vi "Check FETs (Debug).vi"() -> ()   [LabVIEW 2009]
panel:
  out "Debug":string
  out "Emergency Stop":bool=TRUE
  out "Input E":bool=TRUE
  out "Motors on?":bool=TRUE
  out "MC Init Complete":bool=TRUE
  in  "MC VISA resource in":refnum<visa-resource-name>="ASRL1::INSTR"
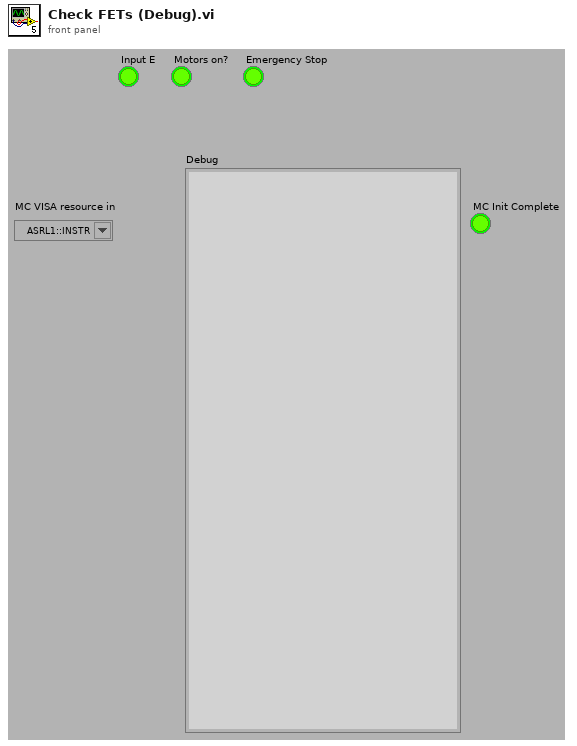
[diagram p1: front panel]
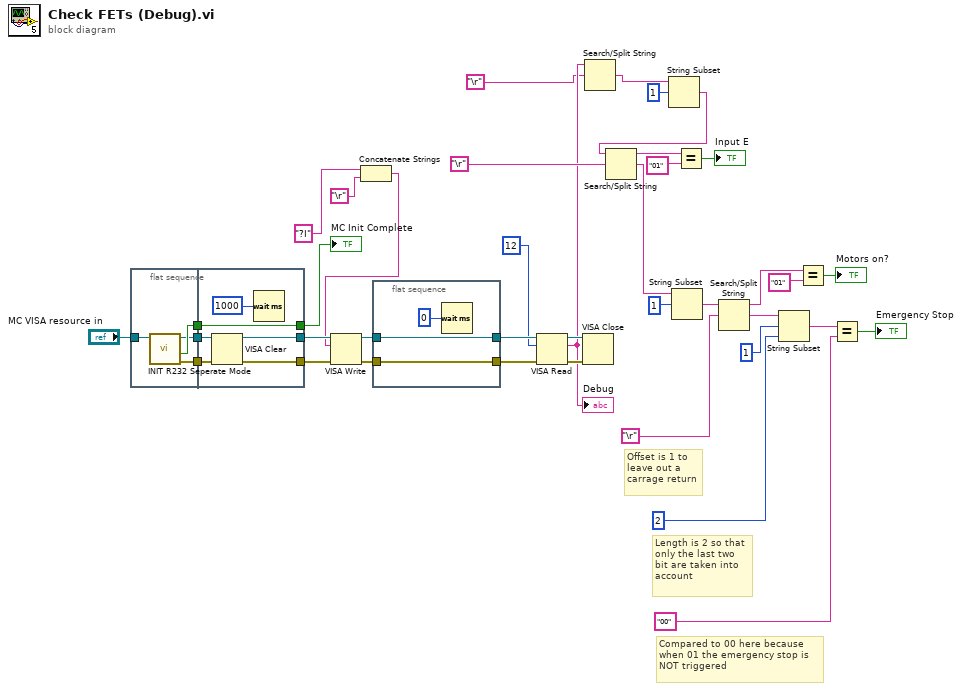
[diagram p0: block diagram]
diagram:
  # "Compared to 00 here because\nwhen 01 the emergency stop is\nNOT triggered"
  # "Length is 2 so that\nonly the last two\nbit are taken into\naccount"
  # "Offset is 1 to\nleave out a\ncarrage return"
  n1 = flat-sequence {
    tunnel: "MC VISA resource in" -> [w43]
    tunnel: [w42] -> w11
    tunnel: [w41] -> w10
    tunnel: [w40] -> w9
    tunnel: [w44] -> w36
    tunnel: [w45] -> w37
    tunnel: [w49] -> w38
    tunnel: w11 -> [w49]
    tunnel: w10 -> [w46]
    tunnel: w9 -> [w47]
    frame #0 {
      n2 = call "INIT R232 Seperate Mode.vi"("MC VISA resource in"=w43) -> ("MC error out"=w40:errorcluster, "MC Init Complete"=w42:bool, "MC VISA resource  out"=w41:refnum<visa-resource-name>)  [unwired: 8 in]
    }
    frame #1 {
      n3 = VISA Clear(VISA resource name=w46, error in (no error)=w47) -> (VISA resource name out=w45:refnum<visa-resource-name>, error out=w44:errorcluster)
      n4 = Wait (ms)(milliseconds to wait=u32 1000) -> ()  [unwired: 1 out]
    }
  }
  n5 = Concatenate Strings("?I" ("write buffer"), "\r") -> (w6:string)
  n6 = VISA Write(VISA resource name=w37, write buffer=w6, error in (no error)=w36) -> (VISA resource name out=w33:refnum<visa-resource-name>, error out=w31:errorcluster)  [unwired: 1 out]
  n7 = flat-sequence {
    tunnel: w33 -> [w52]
    tunnel: [w52] -> w32
    tunnel: w31 -> [w51]
    tunnel: [w51] -> w30
    frame #0 {
      n8 = Wait (ms)(milliseconds to wait=u32 0) -> ()  [unwired: 1 out]
    }
  }
  n9 = VISA Read(VISA resource name=w32, byte count=u32 12, error in (no error)=w30) -> (VISA resource name out=w35:refnum<visa-resource-name>, read buffer=w5:string, error out=w34:errorcluster)  [unwired: 1 out]
  "Debug" <- w5
  n10 = VISA Close(VISA resource name=w35, error in (no error)=w34) -> ()  [unwired: 1 out]
  n11 = Search/Split String(string=w5, search string/char (-)="\r") -> (match + rest of string=w3:string)  [unwired: 1 in, 2 out]
  n12 = String Subset(string=w3, offset (0)=1) -> (substring=w1:string)  [unwired: 1 in]
  n13 = Search/Split String(string=w1, search string/char (-)="\r") -> (substring before match=w28:string, match + rest of string=w25:string)  [unwired: 1 in, 1 out]
  n14 = String Subset(string=w25, offset (0)=1) -> (substring=w23:string)  [unwired: 1 in]
  n15 = Equal?(x=w28, y="01") -> (x = y?=→"Input E":bool)
  n16 = Search/Split String(string=w23, search string/char (-)="\r") -> (substring before match=w21:string, match + rest of string=w18:string)  [unwired: 1 in, 1 out]
  n17 = String Subset(string=w18, offset (0)=1, length (rest)=2 ("length (rest)")) -> (substring=w15:string)
  n18 = Equal?(x=w21, y="01") -> (x = y?=→"Motors on?":bool)
  n19 = Equal?(x=w15, y="00") -> (x = y?=→"Emergency Stop":bool)
  "MC Init Complete" <- w38
